vi "Add Named Attribute Text Element.vi"(6 "Name":string, 7 "Tag Name":string="CodeDocumentation", 8 "error in":errorcluster, 9 "Value":string, 10 "Element in":refnum<k20>, 11 "Document in":refnum<k20>) -> (0 "error out":errorcluster, 2 "Element out":refnum<k20>, 3 "Document out":refnum<k20>)   [LabVIEW 2025]
uses:
  <resource>/objmgr/DOMUserDefRef.rc
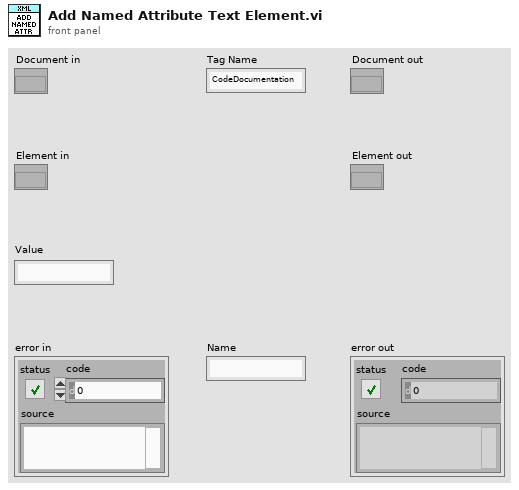
[diagram p1: front panel]
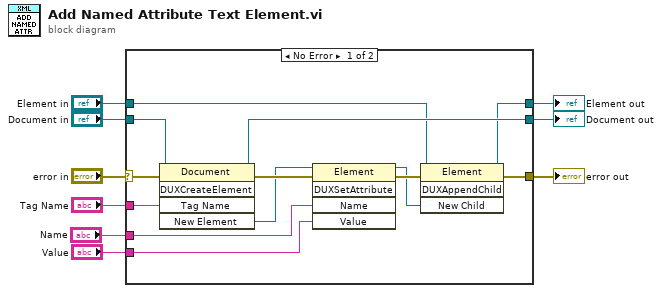
[diagram p0: block diagram]
diagram:
  n1 = case shown="No Error" "error in" {
    selector: "error in" -> [w12 w23]
    tunnel: "Tag Name" -> [w20 _]
    tunnel: "Value" -> [w11 _]
    tunnel: "Document in" -> [w16 w24]
    tunnel: "Element in" -> [w15 w25]
    tunnel: [w19 w24] -> w5
    tunnel: [w14 w25] -> w4
    tunnel: [w13 w23] -> w3
    tunnel: "Name" -> [w10 _]
    frame No Error {
      n2 = invoke class="Document" method="DUXCreateElement"(reference=w16, error in=w12, "Tag Name"=w20) -> (reference out=w19:refnum<k20>, error out=w22:errorcluster, "New Element"=w18:refnum<k20>)  [unwired: 2 in, 2 out]
      n3 = invoke class="Element" method="DUXSetAttribute"(reference=w18, error in=w22, "Name"=w10, "Value"=w11) -> (reference out=w17:refnum<k20>, error out=w21:errorcluster)  [unwired: 1 in, 3 out]
      n4 = invoke class="Element" method="DUXAppendChild"(reference=w15, error in=w21, "New Child"=w17) -> (reference out=w14:refnum<k20>, error out=w13:errorcluster)  [unwired: 1 in, 2 out]
    }
    frame Error {
    }
  }
  "error out" <- w3
  "Document out" <- w5
  "Element out" <- w4
